vi "Update All Timestamps to System Clock.vi"(8 "error in":errorcluster, 9 "ClockID":u8, 10 "Clock Convert Map in":T1, 11 "Bytes in":u8[](array[numeric])) -> (0 "error out":errorcluster, 2 "Records":i32, 3 "Bytes out":u8[](array[numeric]))   [LabVIEW 2021, in "pcap_Parse_Build_CIF.lvclass"]
doc: "Update all timestamps in the pcap bytestream. This will automatically detect if a global header is present and will work on both full pcap streams to/from disk and pcap packets to/from FIFO. If no global header is found it will default to CIF channel format (little endian, ns timestamp)."
uses:
  pcap_Parse_Build_CIF.lvclass
  <vilib>/CIF Foundation/CIF Utilities/Time/Typedef/Clock Conversion Map.ctl
  <vilib>/CIF Foundation/CIF Utilities/Time/Typedef/Timestamp Pair.ctl
  pcap_Parse_Build_CIF.lvclass/pcap_Parse_Build_CIF.ctl
  Add Error.vi
  <vilib>/CIF Foundation/CIF Utilities/DataTypes/Flatten Unflatten/Unflatten U32.vi
  Build/SubVIs/Flatten Packet Header.vi
  <vilib>/CIF Foundation/CIF Utilities/Time/SubVIs/Add Error.vi
  <vilib>/CIF Foundation/CIF Utilities/Errors/Append Error Location.vi
  <vilib>/CIF Foundation/CIF Utilities/DataTypes/Flatten Unflatten/Flatten U32.vi
  <vilib>/CIF Foundation/CIF Utilities/Time/Time_CIF_U.lvlib
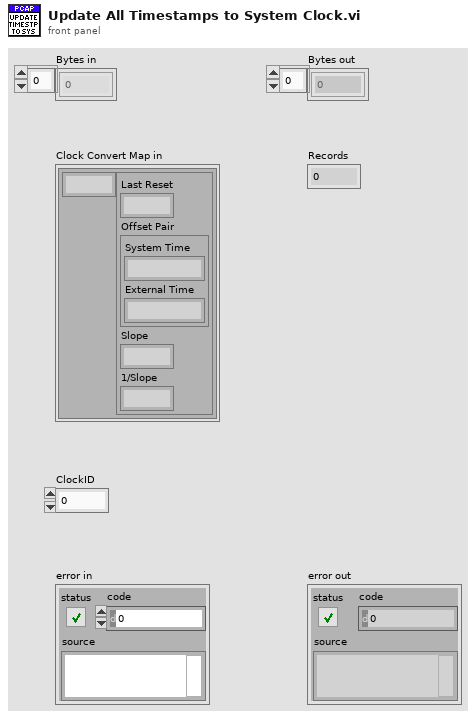
[diagram p1: front panel]
types:
  T1 = typedef "Time_CIF_U.lvlib/Clock Conversion Map.ctl" = map{u8, cluster{"Last Reset":i64, "Offset Pair":T2, "Slope":dbl, "1/Slope":dbl}}
  T2 = typedef "Time_CIF_U.lvlib/Timestamp Pair.ctl" = cluster{"System Time":i64, "External Time":i64}
  T3 = typedef "pcap_Parse_Build_CIF.lvclass/Packet Header.ctl" = cluster{"Timestamp (s)":u32, "Timestamp (ns)":u32, "Inc Length":u32, "Orig Length":u32}
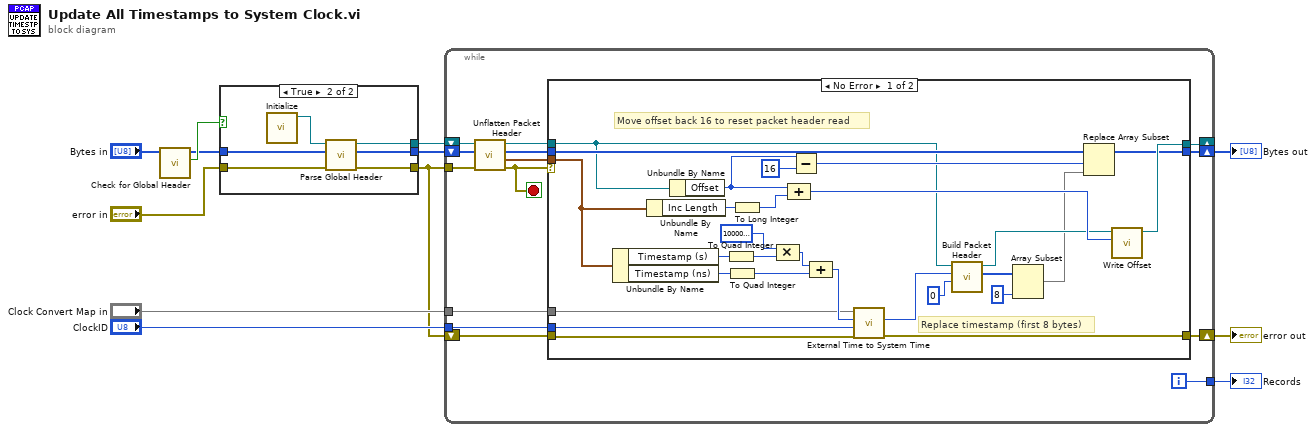
[diagram p0: block diagram]
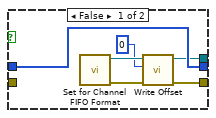
[diagram p3: hidden frame]
diagram:
  n1 = call "Check for Global Header.vi"("Bytes in"="Bytes in") -> ("Global Header Present"=w12:bool, "Bytes out"=w10:u8[])  [unwired: 8 in, 1 out]
  n2 = case shown="True" w12 {
    tunnel: [w14 w20] -> w9
    tunnel: w10 -> [w16 w23]
    tunnel: [w16 w22] -> w11
    tunnel: [w17 w21] -> w4
    tunnel: "error in" -> [_ w18]
    frame False {
      n3 = call "Set for Channel FIFO Format.vi"() -> ("error out"=w17:errorcluster, "pcap_Parse_Build_CIF out"=w15:refnum<class "pcap_Parse_Build_CIF.lvclass">)  [unwired: 10 in]
      n4 = call "Write Offset.vi"("Offset"=0, "pcap Parse and Build in"=w15) -> ("pcap Parse and Build out"=w14:refnum<class "pcap_Parse_Build_CIF.lvclass">)  [unwired: 8 in, 1 out]
    }
    frame True {
      n5 = call "Initialize.vi"() -> ("pcap Parse and Build out"=w19:refnum<class "pcap_Parse_Build_CIF.lvclass">)  [unwired: 11 in]
      n6 = call "Parse Global Header.vi"("error in"=w18, "Bytes in"=w23, "pcap Parse and Build in"=w19) -> ("error out"=w21:errorcluster, "Bytes out"=w22:u8[], "pcap Parse and Build out"=w20:refnum<class "pcap_Parse_Build_CIF.lvclass">)  [unwired: 5 in, 1 out]
    }
  }
  n7 = while {
    tunnel: w4 -> [w36]
    shift-right: [w34] -> _
    shift-left: w9 -> [w35]
    shift-right: [w30] -> w7
    shift-left: w11 -> [w37]
    tunnel: "Clock Convert Map in" -> [w28]
    tunnel: "ClockID" -> [w27]
    shift-right: [w26] -> w2
    shift-left: w4 -> [w25]
    tunnel: [w24] -> w1
    i -> [w24]
    stop <- w29 stop-if-true
    n8 = call "Unflatten Packet Header.vi"("error in (no error)"=w36, "Bytes in"=w37, "pcap Parse and Build in"=w35) -> ("error out"=w29:errorcluster, "Packet Header"=w33:T3, "Bytes out"=w31:u8[], "pcap Parse and Build out"=w32:refnum<class "pcap_Parse_Build_CIF.lvclass">)  [unwired: 5 in]
    n9 = case shown="No Error" w29 {
      tunnel: [w65 w67] -> w34
      tunnel: w33 -> [w63 _]
      tunnel: w32 -> [w48 w67]
      tunnel: w31 -> [w53 w66]
      tunnel: [w51 w66] -> w30
      tunnel: w28 -> [w41 _]
      tunnel: w27 -> [w40 _]
      tunnel: [w39 _] -> w26
      tunnel: w25 -> [w38 _]
      frame No Error {
        # "Replace timestamp (first 8 bytes)"
        # "Move offset back 16 to reset packet header read"
        n10 = Unbundle By Name(w63) -> ("Timestamp (s)"=w60:u32, "Timestamp (ns)"=w59:u32)
        n11 = Unbundle By Name(w63) -> ("Inc Length"=w61:u32)
        n12 = Unbundle By Name(w48) -> ("Offset"=w54:i32)
        n13 = To Quad Integer(1:w60) -> (0:w58:i64)
        n14 = To Quad Integer(1:w59) -> (0:w56:i64)
        n15 = To Long Integer(number=w61) -> (32bit integer=w49:i32)
        n16 = Compound Arithmetic op=MULTIPLY(i64 1000000000 ("x"), w58) -> (w55:i64)
        n17 = Compound Arithmetic op=ADD(w54, w49) -> (w64:i32)
        n18 = Subtract(x=w54, y=16) -> (x-y=w52:i32)
        n19 = Compound Arithmetic op=ADD(w55, w56) -> (w43:i64)
        n20 = call <vilib>:"External Time to System Time.vi"("error in (no error)"=w38, "ClockID"=w40, "External Time"=w43, "Clock Convert Map in"=w41) -> ("error out"=w39:errorcluster, "System Time"=w42:i64)  [unwired: 4 in, 2 out]
        n21 = call "Build Packet Header.vi"("Length"=0, "TAI Time (ns)"=w42, "pcap Parse and Build in"=w48) -> ("Flattened Data out"=w47:u8[], "pcap Parse and Build out"=w50:refnum<class "pcap_Parse_Build_CIF.lvclass">)  [unwired: 7 in]
        n22 = Array Subset(array=w47, length=8) -> (w46:u8[])  [unwired: 1 in]
        n23 = Replace Array Subset(array=w53, new element=w46, index=w52) -> (w51:u8[])
        n24 = call "Write Offset.vi"("Offset"=w64, "pcap Parse and Build in"=w50) -> ("pcap Parse and Build out"=w65:refnum<class "pcap_Parse_Build_CIF.lvclass">)  [unwired: 8 in, 1 out]
      }
      frame Error {
      }
    }
  }
  "Bytes out" <- w7
  "error out" <- w2
  "Records" <- w1
